vi "IsoPlane_Settings.vi"(8 "error in (no error)":errorcluster, 11 "LightField Automation in":refnum<class "LightField Automation.lvclass">) -> (0 "error out":errorcluster, 3 "LightField Automation out":refnum<class "LightField Automation.lvclass">)   [LabVIEW 2018]
uses:
  ProgramData/Documents/Princeton Instruments/LightField/Add-in and Automation SDK/Samples/LabVIEW Automation/lightfield-automation-labview/LightField Automation.lvclass
  C:/Program Files/Princeton Instruments/LightField/PrincetonInstruments.LightFieldAddInSupportServices.dll
  Program Files/Princeton Instruments/LightField/PrincetonInstruments.LightFieldAddInSupportServices.dll
panel:
  in  "OK Button":bool
  in  "Selected grating":string(combo)
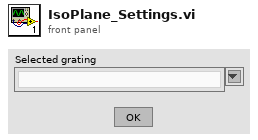
[diagram p1: front panel]
types:
  T1 = cluster{"Parsed Text":string, "GratingSelected":string}[]
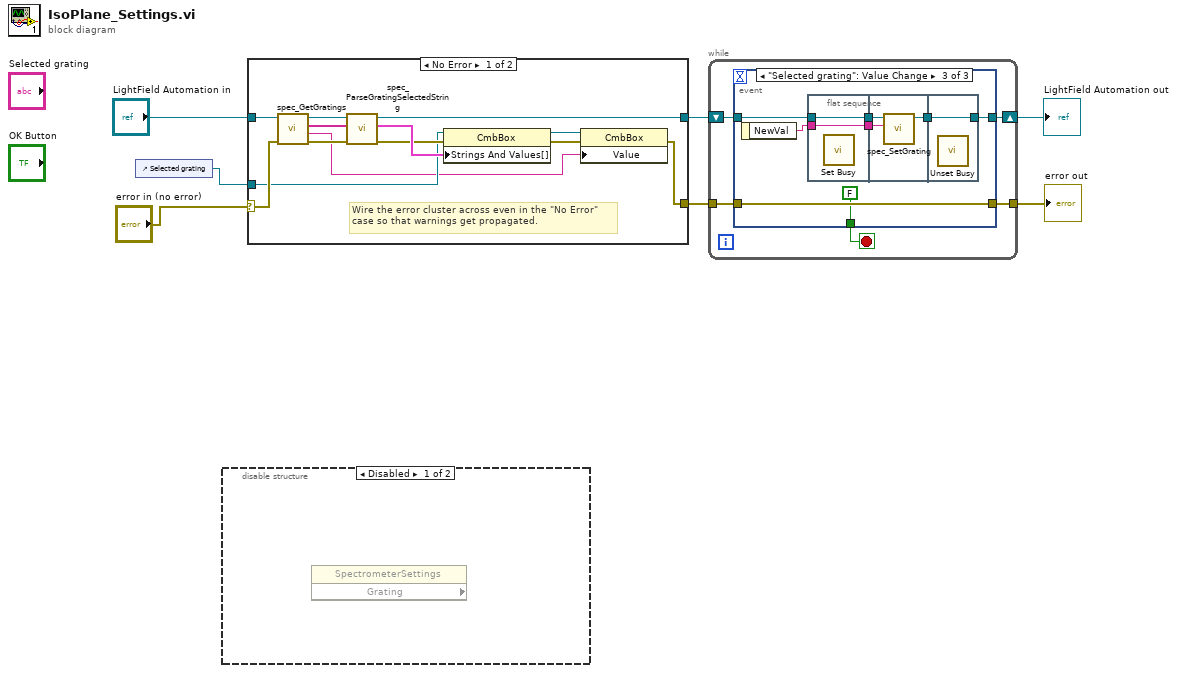
[diagram p0: block diagram]
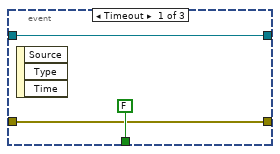
[diagram p2: hidden frame]
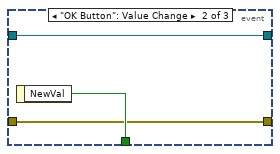
[diagram p3: hidden frame]
diagram:
  n1 = control-ref of="Selected grating"() -> (w7:refnum<vi>)
  n2 = disable-structure shown="Disabled" {
    frame Disabled {
      n3 = property class="SpectrometerSettings" props=["Grating"]() -> ()  [unwired: 2 in, 3 out]
    }
    frame Enabled {
    }
  }
  n4 = case shown="No Error" "error in (no error)" {
    selector: "error in (no error)" -> [w15 w22]
    tunnel: [w8 w22] -> w1
    tunnel: [w16 w21] -> w3
    tunnel: "LightField Automation in" -> [w20 w21]
    tunnel: w7 -> [w12 _]
    frame No Error {
      # "Wire the error cluster across even in the \"No Error\"\ncase so that warnings get propagated."
      n5 = call "spec_GetGratings.vi"("error in (no error)"=w15, "LightField Automation in"=w20) -> ("error out"=w19:errorcluster, "Current Grating"=w9:string, "Gratings"=w18:string[], "LightField Automation out"=w17:refnum<class "LightField Automation.lvclass">)  [unwired: 6 in]
      n6 = call "spec_ParseGratingSelectedString.vi"("error in (no error)"=w19, "GratingsSelected"=w18, "LightField Automation in"=w17) -> ("error out"=w13:errorcluster, "Strings and Values Array"=w14:T1, "LightField Automation out"=w16:refnum<class "LightField Automation.lvclass">)  [unwired: 6 in]
      n7 = property class="CmbBox"(reference=w12, error in=w13, "Strings And Values[]"=w14) -> (reference out=w11:refnum<vi>, error out=w10:errorcluster)
      n8 = property class="CmbBox"(reference=w11, error in=w10, "Value"=w9) -> (error out=w8:errorcluster)  [unwired: 1 out]
    }
    frame Error {
    }
  }
  n9 = while {
    tunnel: [w24] -> w2
    tunnel: w1 -> [w23]
    shift-right: [w26] -> w4
    shift-left: w3 -> [w25]
    stop <- w27 stop-if-true
    n10 = event shown="[2] \"Selected grating\": Value Change" {
      selector: _ -> [_ _ _]
      dyn-events: _ -> [_ _ _]
      timeout: _ -> [_ _ _]
      tunnel: [FALSE ("NewVal") w33 FALSE ("NewVal")] -> w27
      tunnel: [w28 w31 w37] -> w26
      tunnel: w25 -> [w28 w31 w38]
      tunnel: [w29 w32 w41] -> w24
      tunnel: w23 -> [w29 w32 w41]
      event Timeout {
        n11 = event-data() -> ()  [unwired: 1 in, 3 out]
      }
      event "OK Button": Value Change {
        n12 = event-data() -> ("NewVal"=w33:bool)  [unwired: 1 in]
      }
      event "Selected grating": Value Change {
        n13 = event-data() -> ("NewVal"=w39:string)  [unwired: 1 in]
        n14 = flat-sequence {
          tunnel: w38 -> [w42]
          tunnel: w39 -> [w43]
          tunnel: [w43] -> w35
          tunnel: [w42] -> w34
          tunnel: [w44] -> w36
          tunnel: w35 -> [w46]
          tunnel: w34 -> [w45]
          tunnel: [w47] -> w37
          tunnel: w36 -> [w47]
          frame #0 {
            n15 = call <vilib>:"Set Busy.vi"() -> ()  [unwired: 10 in, 2 out]
          }
          frame #1 {
            n16 = call "spec_SetGrating.vi"("GratingSelected"=w46, "LightField Automation in"=w45) -> ("LightField Automation out"=w44:refnum<class "LightField Automation.lvclass">)  [unwired: 8 in, 1 out]
          }
          frame #2 {
            n17 = call <vilib>:"Unset Busy.vi"() -> ()  [unwired: 11 in, 1 out]
          }
        }
      }
    }
  }
  "error out" <- w2
  "LightField Automation out" <- w4
